vi "channels_settings.vi"(7 "Mode":u32(ring) items=["Unknown", "Trig", "Stream"], 8 "error in (no error)":errorcluster, 9 "Sampling Frequency":dbl, 10 "Bits":u8(slide)=12 min=12 max=16 step=2 scale=12.0..16.0, 11 "SCP_id":u32) -> (0 "error out":errorcluster, 2 "Fs":dbl, 3 "OSC_ID":u32)   [LabVIEW 2018]
uses:
  LibTiePie.lvlib
  LabViewHS4/libtiepie.dll
panel:
  out "Resolution":u8
  out "MeasureMode":u32
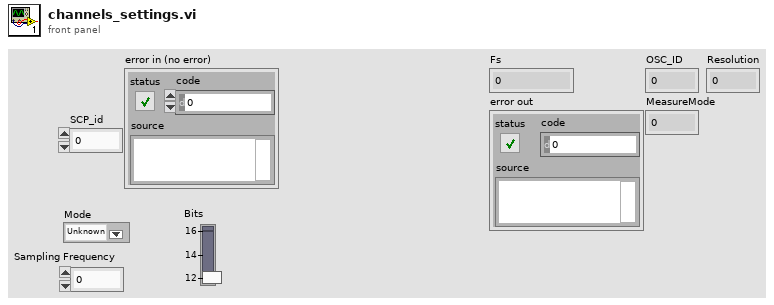
[diagram p1: front panel]
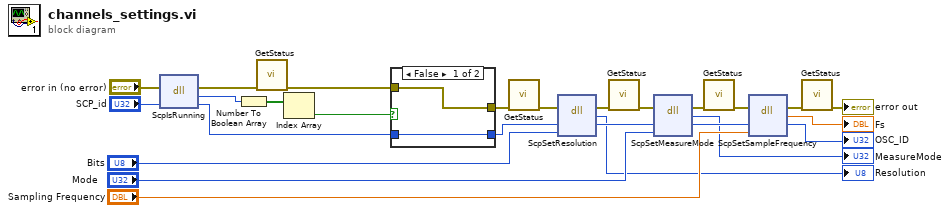
[diagram p0: block diagram]
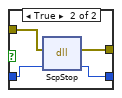
[diagram p2: hidden frame]
diagram:
  n1 = dll-call lib="C:/Users/cwaha/Documents/LabViewHS4/libtiepie.dll" fn="ScpIsRunning"(error in="error in (no error)", "ScpHandle"="SCP_id") -> (error out=w9:errorcluster, "isRunning"=w6:u8, "ScpHandle"=w7:u32)  [unwired: 2 in, 1 out]
  n2 = Number To Boolean Array(number=w6) -> (Boolean array=w5:bool[])
  n3 = call "GetStatus.vi"("error in (no error)"=w9) -> ("error out"=w11:errorcluster)  [unwired: 10 in]
  n4 = Index Array(array=w5) -> (element=w4:bool)  [unwired: 1 in]
  n5 = case shown="False" w4 {
    tunnel: w7 -> [w27 w32]
    tunnel: w11 -> [w28 w31]
    tunnel: [w28 w30] -> w26
    tunnel: [w27 w29] -> w12
    frame False {
    }
    frame True {
      n6 = dll-call lib="C:/Users/cwaha/Documents/LabViewHS4/libtiepie.dll" fn="ScpStop"(error in=w31, "SCP_ID"=w32) -> (error out=w30:errorcluster, "SCP_ID"=w29:u32)  [unwired: 3 in, 1 out]
    }
  }
  n7 = call "GetStatus.vi"("error in (no error)"=w26) -> ("error out"=w25:errorcluster)  [unwired: 10 in]
  n8 = dll-call lib="C:/Users/cwaha/Documents/LabViewHS4/libtiepie.dll" fn="ScpSetResolution"(error in=w25, "SCP_id"=w12, "RES"="Bits") -> (error out=w24:errorcluster, "return type"=→"Resolution":u8, "SCP_id"=w21:u32)  [unwired: 3 in, 1 out]
  n9 = call "GetStatus.vi"("error in (no error)"=w24) -> ("error out"=w23:errorcluster)  [unwired: 10 in]
  n10 = dll-call lib="C:/Users/cwaha/Documents/LabViewHS4/libtiepie.dll" fn="ScpSetMeasureMode"(error in=w23, "SCP_ID"=w21, "MeasureMode"="Mode") -> (error out=w20:errorcluster, "return type"=→"MeasureMode":u32, "SCP_ID"=w18:u32)  [unwired: 3 in, 1 out]
  n11 = call "GetStatus.vi"("error in (no error)"=w20) -> ("error out"=w19:errorcluster)  [unwired: 10 in]
  n12 = dll-call lib="C:/Users/cwaha/Documents/LabViewHS4/libtiepie.dll" fn="ScpSetSampleFrequency"(error in=w19, "OSC_ID"=w18, "FS"="Sampling Frequency") -> (error out=w15:errorcluster, "FS_out"=→"Fs":dbl, "OSC_ID"=→"OSC_ID":u32)  [unwired: 3 in, 1 out]
  n13 = call "GetStatus.vi"("error in (no error)"=w15) -> ("error out"=→"error out":errorcluster)  [unwired: 10 in]
